vi "Ballard XML Generator.Add Hardware Channel.vi"(10 "channel":i32, 11 "string in":string) -> (3 "string out":string)   [LabVIEW 2017]
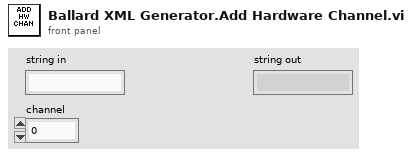
[diagram p1: front panel]
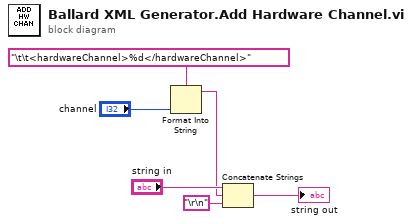
[diagram p0: block diagram]
diagram:
  n1 = Format Into String(format string="\t\t<hardwareChannel>%d</hardwareChannel>", "channel") -> (resulting string=w2:string)  [unwired: 2 in, 1 out]
  n2 = Concatenate Strings("string in", w2, "\r\n") -> (→"string out":string)
